vi "Day 4.vi"() -> ()   [LabVIEW 2021]
panel:
  out "input":string
  out "input file":path
  out "ouptut 2":i16
  in  "Run [T]/ Example[F]":bool
  out "ouptut 1":i16
  # "Advent of Code 2022 - Day 4 - Camp Cleanup"
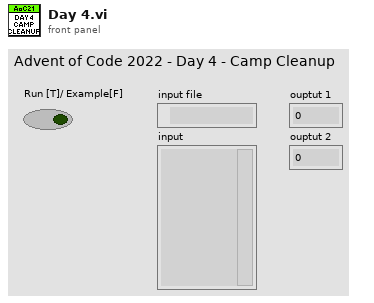
[diagram p1: front panel]
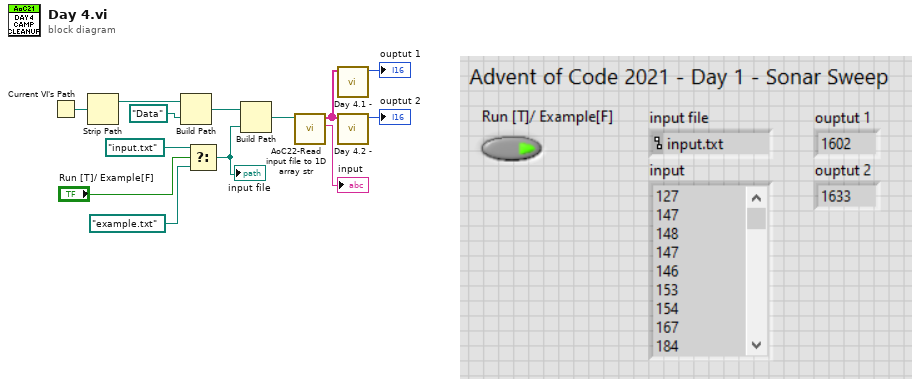
[diagram p0: block diagram]
diagram:
  n1 = Current VI's Path() -> (path=w13:path)
  n2 = Strip Path(path=w13) -> (stripped path=w11:path)  [unwired: 1 out]
  n3 = Build Path(base path=w11, name or relative path=path "Data") -> (appended path=w9:path)
  n4 = Select(t=path "input.txt" ("name or relative path"), s="Run [T]/ Example[F]", f=path "example.txt" ("name or relative path")) -> (s? t:f=w5:path)
  "input file" <- w5
  n5 = Build Path(base path=w9, name or relative path=w5) -> (appended path=w12:path)
  n6 = call "AoC22-Read input file to 1D array str.vi"("input file"=w12) -> ("input text"=→"input":string, "input"=w1:string[])  [unwired: 9 in]
  n7 = call "Day 4.1 - .vi"("input"=w1) -> ("output"=→"ouptut 1":i16)  [unwired: 10 in]
  n8 = call "Day 4.2 - .vi"("input"=w1) -> ("output"=→"ouptut 2":i16)  [unwired: 10 in]
